vi "Clide Tele-Op.vi"(8 "Operator Buttons":bool[](array[boolean]), 9 "Operator Axes":dbl[](array[numeric]), 10 "Driver Buttons":bool[](array[boolean]), 11 "Driver Axes":dbl[](array[numeric])) -> ()   [LabVIEW 2019]
uses:
  Implementation/Clide Operations.ctl
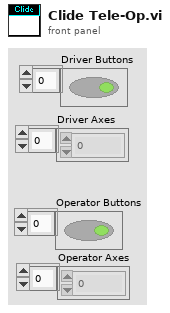
[diagram p1: front panel]
types:
  T1 = typedef "Clide Operations.ctl" = enum16{"Reserve", "Read Current", "Immediate", "Color Wheel"}
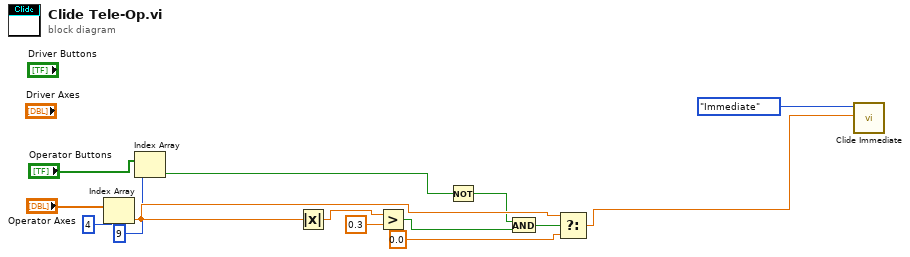
[diagram p0: block diagram]
diagram:
  n1 = Index Array(array="Operator Axes", index=4) -> (element=w8:dbl)
  n2 = Index Array(array="Operator Buttons", index=9) -> (element=w1:bool)
  n3 = Absolute Value(x=w8) -> (abs(x)=w7:dbl)
  n4 = Greater?(x=w7, y=0.3) -> (0:w5:bool)
  n5 = Not(x=w1) -> (.not. x?=w2:bool)
  n6 = And(x=w2, y=w5) -> (x .and. y?=w6:bool)
  n7 = Select(t=w8, s=w6, f=0.0) -> (s? t:f=w9:dbl)
  n8 = call "Clide Immediate.vi"("Power"=w9, "Operation"=Clide_Operations."Immediate") -> ()  [unwired: 10 in]
